vi "Generate_Clear_Errors.vi"(8 "error in (no error)":errorcluster, 9 "location":T1, 11 "VI in":refnum<vi>) -> (0 "error out":errorcluster, 1 "error out term":refnum<vi>, 2 "error in term":refnum<vi>, 3 "object refnum":refnum<vi>)   [LabVIEW 2025]
uses:
  <vilib>/Utility/miscctls.llb/LVPointTypeDef.ctl
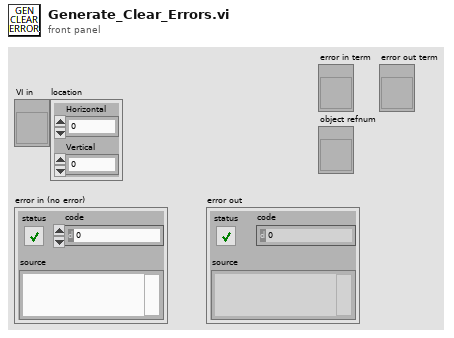
[diagram p1: front panel]
types:
  T1 = typedef "LVPointTypeDef.ctl" = cluster{"Horizontal":i16, "Vertical":i16}
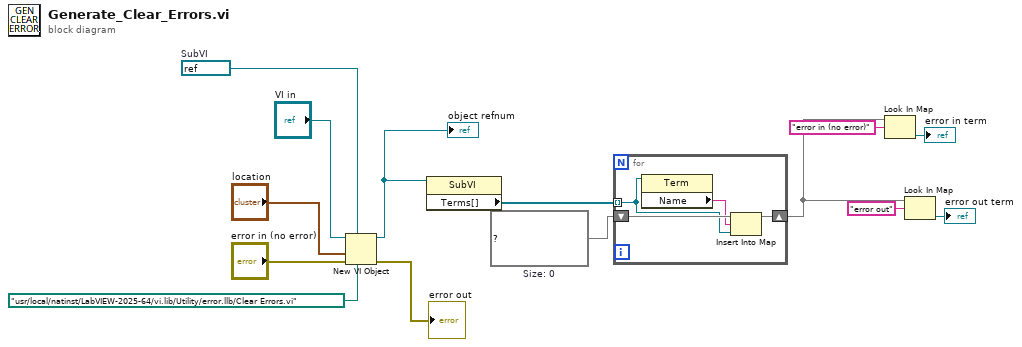
[diagram p0: block diagram]
diagram:
  w7 = map{string, refnum<vi>} {}  # Size: 0
  w14 = refnum<vi> refnum  # SubVI
  n1 = New VI Object(vi object class=w14, owner refnum="VI in", position/next to="location", 6:path "/usr/local/natinst/LabVIEW-2025-64/vi.lib/Utility/error.llb/Clear Errors.vi" ("path"), 8:"error in (no error)") -> (object refnum=w8:refnum<vi>, 0:→"error out":errorcluster)  [unwired: 3 in]
  "object refnum" <- w8
  n2 = property class="SubVI"(reference=w8) -> ("Terms[]"=w6:refnum<vi>[])  [unwired: 1 in, 2 out]
  n3 = for {
    tunnel: w6 -> [w15] mode=indexing
    shift-right: [w17] -> w3
    shift-left: w7 -> [w18]
    n4 = property class="Term"(reference=w15) -> ("Name"=w16:string)  [unwired: 1 in, 2 out]
    n5 = Insert Into Map(map in=w18, key=w16, value=w15) -> (map out=w17:map{string, refnum<vi>})  [unwired: 2 out]
  }
  n6 = Look In Map(map=w3, key="error in (no error)") -> (value=→"error in term":refnum<vi>)  [unwired: 1 in, 1 out]
  n7 = Look In Map(map=w3, key="error out") -> (value=→"error out term":refnum<vi>)  [unwired: 1 in, 1 out]
